vi "Launch PID Loop.vi"(8 "error in (no error)":errorcluster, 11 "PID Loop":refnum<class "PID Loop.lvclass">) -> (0 "error out":errorcluster, 2 "PID Notifiers":T1, 3 "Message Queue out":refnum<queue>)   [LabVIEW 2024, in "PID Loop.lvlib" / "PID Loop.lvclass"]
uses:
  PID Loop.lvclass
  PID Loop.lvclass/PID Loop.ctl
  src/Zero Timeout Message Handler/Zero Timeout Message Handler/Zero Timeout Message Handler.lvclass
  Get Notifiers Msg/Get Notifiers Msg.lvclass
  src/Zero Timeout Message Handler/~Message/~Message.lvclass
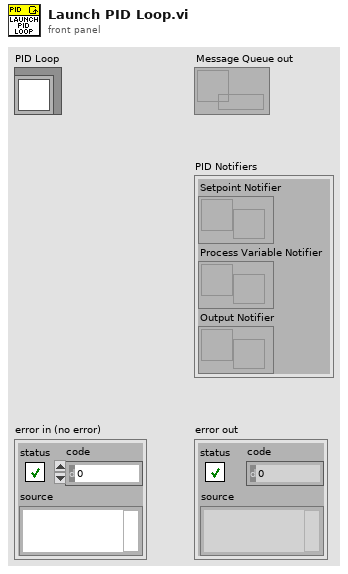
[diagram p1: front panel]
types:
  T1 = cluster{"Setpoint Notifier":refnum<notifier>, "Process Variable Notifier":refnum<notifier>, "Output Notifier":refnum<notifier>}
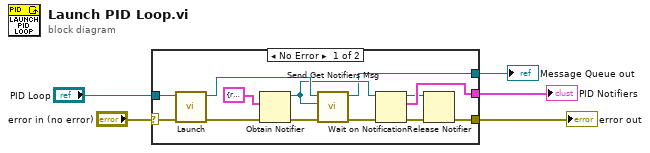
[diagram p0: block diagram]
diagram:
  n1 = case shown="No Error" "error in (no error)" {
    selector: "error in (no error)" -> [w7 w19]
    tunnel: "PID Loop" -> [w18 _]
    tunnel: [w11 _] -> w4
    tunnel: [w8 w19] -> w3
    tunnel: [w6 _] -> w1
    frame No Error {
      n2 = call "Launch.vi"("error in (no error)"=w7, "Zero Timeout Message Handler in"=w18) -> ("error out"=w15:errorcluster, "Message Queue"=w17:refnum<queue>)  [unwired: 8 in]
      n3 = Obtain Notifier(notification data type=T1 {"Setpoint Notifier"=refnum, "Process Variable Notifier"=refnum, "Output Notifier"=refnum} ("notification"), error in (no error)=w15) -> (notifier out=w12:refnum<notifier>, error out=w14:errorcluster)  [unwired: 2 in, 1 out]
      n4 = call "Send Get Notifiers Msg.vi"("error in (no error)"=w14, "Notifier of Notifiers"=w12, "Message Queue in"=w17) -> ("error out"=w13:errorcluster, "Message Queue out"=w6:refnum<queue>)  [unwired: 7 in]
      n5 = Wait on Notification(notifier=w12, error in (no error)=w13) -> (notifier out=w10:refnum<notifier>, notification=w11:T1, error out=w9:errorcluster)  [unwired: 2 in, 1 out]
      n6 = Release Notifier(notifier=w10, error in (no error)=w9) -> (error out=w8:errorcluster)  [unwired: 1 in, 2 out]
    }
    frame Error {
    }
  }
  "error out" <- w3
  "PID Notifiers" <- w4
  "Message Queue out" <- w1
